vi "Extract All UI Strings.vi"(8 "error in (no error)":errorcluster, 9 "Config (All)":T1={"FP Decoration Text"=TRUE, "FP Controls"=TRUE, "BD Text"=TRUE}, 11 "LanguageData in":refnum<class "VI Data.lvclass">) -> (0 "error out":errorcluster, 3 "LanguageData out":refnum<class "VI Data.lvclass">)   [LabVIEW 2013, in "SET Project Data.lvlib" / "VI Data.lvclass"]
uses:
  VI Data.lvclass
  VI Data.lvclass/VI Data.ctl
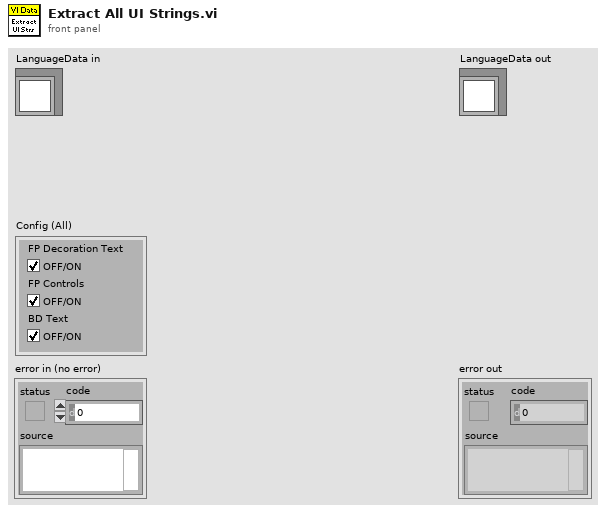
[diagram p1: front panel]
types:
  T1 = cluster{"FP Decoration Text":bool, "FP Controls":bool, "BD Text":bool}
  T2 = enum32{"invalid VI type", "Standard VI", "Control VI", "Global VI", "Polymorphic VI", "Configuration VI", "SubSystem", "Facade VI", "Method VI", "Statechart Diagram VI"}
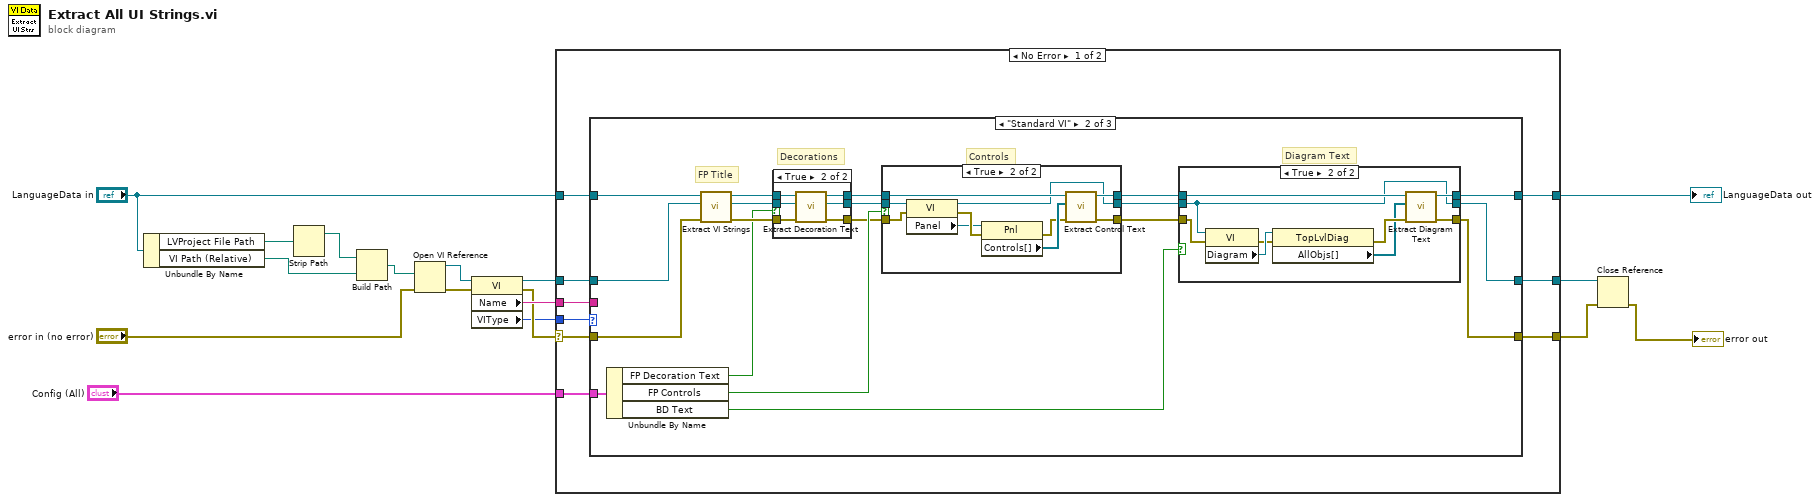
[diagram p0: block diagram]
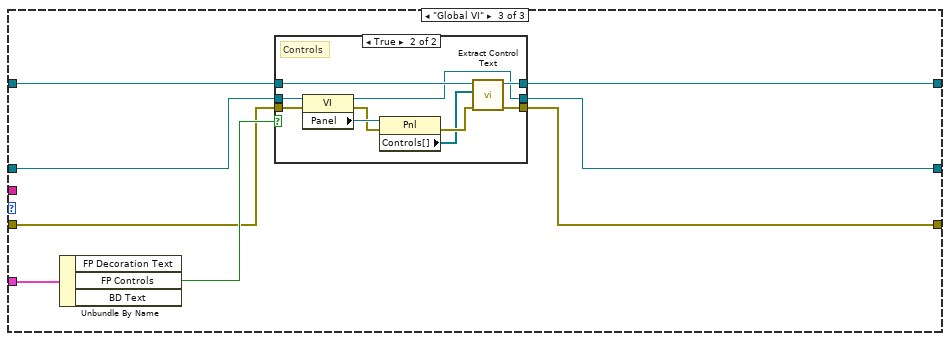
[diagram p6: hidden frame]
diagram:
  n1 = Unbundle By Name("LanguageData in") -> ("LVProject File Path"=w2:path, "VI Path (Relative)"=w5:path)
  n2 = Strip Path(path=w2) -> (stripped path=w3:path)  [unwired: 1 out]
  n3 = Build Path(base path=w3, name or relative path=w5) -> (appended path=w4:path)
  n4 = Open VI Reference(vi path=w4, error in (no error)="error in (no error)") -> (vi reference=w15:refnum<vi>, error out=w14:errorcluster)  [unwired: 4 in]
  n5 = property class="VI"(reference=w15, error in=w14) -> (reference out=w13:refnum<vi>, error out=w10:errorcluster, "Name"=w12:string, "VIType"=w1:T2)
  n6 = case shown="No Error" w10 {
    selector: w10 -> [w19 w105]
    tunnel: [w25 w105] -> w8
    tunnel: [w26 w106] -> w17
    tunnel: "LanguageData in" -> [w23 w106]
    tunnel: "Config (All)" -> [w24 _]
    tunnel: w13 -> [w20 w104]
    tunnel: w12 -> [w22 _]
    tunnel: [w21 w104] -> w9
    tunnel: w1 -> [w18 _]
    frame No Error {
      n7 = case shown="\"Standard VI\"" w18 {
        tunnel: [w27 w32 w83] -> w26
        tunnel: [w28 w31 w84] -> w25
        tunnel: w24 -> [_ w48 w90]
        tunnel: w23 -> [w27 w46 w86]
        tunnel: w22 -> [_ _ _]
        tunnel: [w29 w30 w85] -> w21
        tunnel: w20 -> [w29 w45 w87]
        tunnel: w19 -> [w28 w44 w88]
        frame "invalid VI type", Default {
        }
        frame "Standard VI" {
          # "Controls"
          # "FP Title"
          # "Diagram Text"
          # "Decorations"
          n8 = Unbundle By Name(w48) -> ("FP Decoration Text"=w40:bool, "FP Controls"=w39:bool, "BD Text"=w47:bool)
          n9 = call "Extract VI Strings.vi"("SET VI in"=w46, "VI Ref in"=w45, "error in (no error)"=w44) -> ("SET VI out"=w43:refnum<class "VI Data.lvclass">, "VI Ref out"=w42:refnum<vi>, "error out"=w41:errorcluster)  [unwired: 5 in]
          n10 = case shown="True" w40 {
            tunnel: [w64 w69] -> w38
            tunnel: w41 -> [w64 w70]
            tunnel: w42 -> [w62 w68]
            tunnel: [w62 w67] -> w36
            tunnel: w43 -> [w63 w66]
            tunnel: [w63 w65] -> w37
            frame False {
            }
            frame True {
              n11 = call "Extract Decoration Text.vi"("error in (no error)"=w70, "VI Ref in"=w68, "VI Data in"=w66) -> ("error out"=w69:errorcluster, "VI Ref out"=w67:refnum<vi>, "VI Data out"=w65:refnum<class "VI Data.lvclass">)  [unwired: 6 in]
            }
          }
          n12 = case shown="True" w39 {
            tunnel: w38 -> [w49 w55]
            tunnel: w37 -> [w51 w61]
            tunnel: w36 -> [w50 w58]
            tunnel: [w51 w54] -> w33
            tunnel: [w49 w53] -> w35
            tunnel: [w50 w52] -> w34
            frame False {
            }
            frame True {
              n13 = property class="VI"(reference=w58, error in=w55) -> (reference out=w52:refnum<vi>, error out=w60:errorcluster, "Panel"=w59:refnum<vi>)
              n14 = property class="Pnl"(reference=w59, error in=w60) -> (error out=w56:errorcluster, "Controls[]"=w57:refnum<vi>[])  [unwired: 1 out]
              n15 = call "Extract Control Text.vi"("error in (no error)"=w56, "ControlRefs[]"=w57, "VI Data in"=w61) -> ("error out"=w53:errorcluster, "VI Data out"=w54:refnum<class "VI Data.lvclass">)  [unwired: 7 in]
            }
          }
          n16 = case shown="True" w47 {
            tunnel: [w73 w77] -> w31
            tunnel: w35 -> [w73 w80]
            tunnel: w34 -> [w71 w74]
            tunnel: w33 -> [w72 w76]
            tunnel: [w72 w75] -> w32
            tunnel: [w71 w74] -> w30
            frame False {
            }
            frame True {
              n17 = property class="VI"(reference=w74, error in=w80) -> (error out=w81:errorcluster, "Diagram"=w82:refnum<vi>)  [unwired: 1 out]
              n18 = property class="TopLvlDiag"(reference=w82, error in=w81) -> (error out=w79:errorcluster, "AllObjs[]"=w78:refnum<vi>[])  [unwired: 1 out]
              n19 = call "Extract Diagram Text.vi"("error in (no error)"=w79, "DiagObjRefs[]"=w78, "VI Data in"=w76) -> ("error out"=w77:errorcluster, "VI Data out"=w75:refnum<class "VI Data.lvclass">)  [unwired: 7 in]
            }
          }
        }
        frame "Global VI" {
          n20 = Unbundle By Name(w90) -> ("FP Controls"=w89:bool)  [unwired: 2 out]
          n21 = case shown="True" w89 {
            tunnel: [w93 w99] -> w84
            tunnel: w88 -> [w93 w101]
            tunnel: w87 -> [w92 w97]
            tunnel: w86 -> [w91 w96]
            tunnel: [w91 w95] -> w83
            tunnel: [w92 w94] -> w85
            frame False {
            }
            frame True {
              # "Controls"
              n22 = property class="VI"(reference=w97, error in=w101) -> (reference out=w94:refnum<vi>, error out=w102:errorcluster, "Panel"=w103:refnum<vi>)
              n23 = property class="Pnl"(reference=w103, error in=w102) -> (error out=w100:errorcluster, "Controls[]"=w98:refnum<vi>[])  [unwired: 1 out]
              n24 = call "Extract Control Text.vi"("error in (no error)"=w100, "ControlRefs[]"=w98, "VI Data in"=w96) -> ("error out"=w99:errorcluster, "VI Data out"=w95:refnum<class "VI Data.lvclass">)  [unwired: 7 in]
            }
          }
        }
      }
    }
    frame Error {
    }
  }
  "LanguageData out" <- w17
  n25 = Close Reference(reference=w9, error in (no error)=w8) -> (error out=→"error out":errorcluster)
